vi "CalculatePattern.vi"(4 "Patterns":T2, 5 "error in (no error)":errorcluster, 6 "Colour Set":T1, 8 "NeoPixel Ring in":T1) -> (0 "error out":errorcluster, 2 "NeoPixel Ring out":T1)   [LabVIEW 2020, in "CTI-Scratchpad.lvlib"]
uses:
  CTI-Scratchpad.lvlib
  NeoPixelRingPatterns.ctl
panel:
  # "Input"
  # "Output"
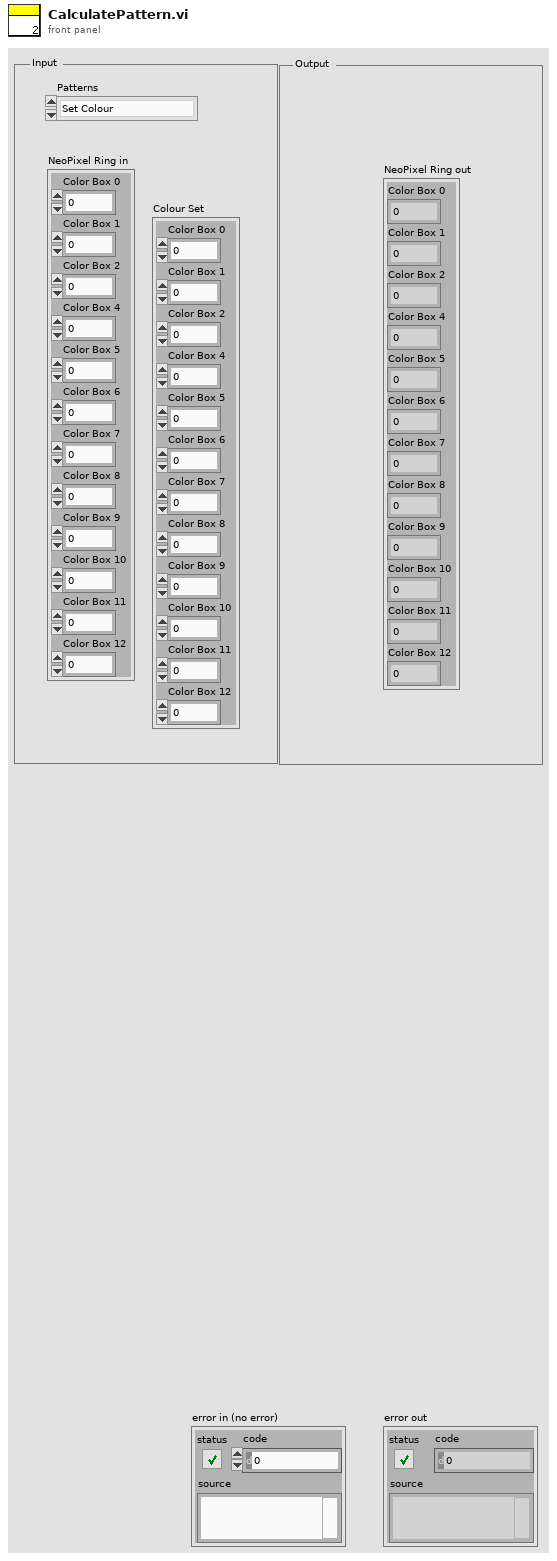
[diagram p1: front panel]
types:
  T1 = cluster{"Color Box 0":u32, "Color Box 1":u32, "Color Box 2":u32, "Color Box 4":u32, "Color Box 5":u32, "Color Box 6":u32, "Color Box 7":u32, "Color Box 8":u32, "Color Box 9":u32, "Color Box 10":u32, "Color Box 11":u32, "Color Box 12":u32}
  T2 = typedef "CTI-Scratchpad.lvlib/NeoPixelRingPatterns.ctl" = enum16{"Set Colour", "ColorWipe", "TheatreChase", "Rainbow"}
  T3 = cluster{"[0]":u32, "[1]":u32, "[2]":u32, "[3]":u32, "[4]":u32, "[5]":u32, "[6]":u32, "[7]":u32, "[8]":u32, "[9]":u32, "[10]":u32, "[11]":u32}
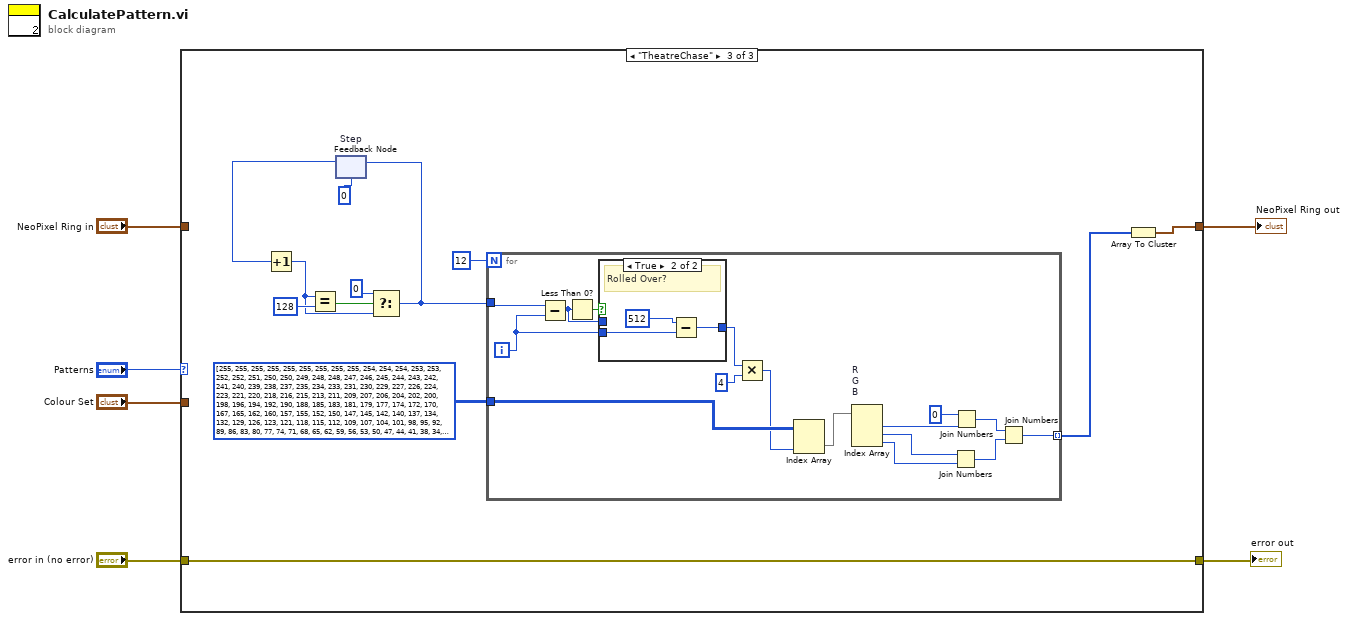
[diagram p0: block diagram]
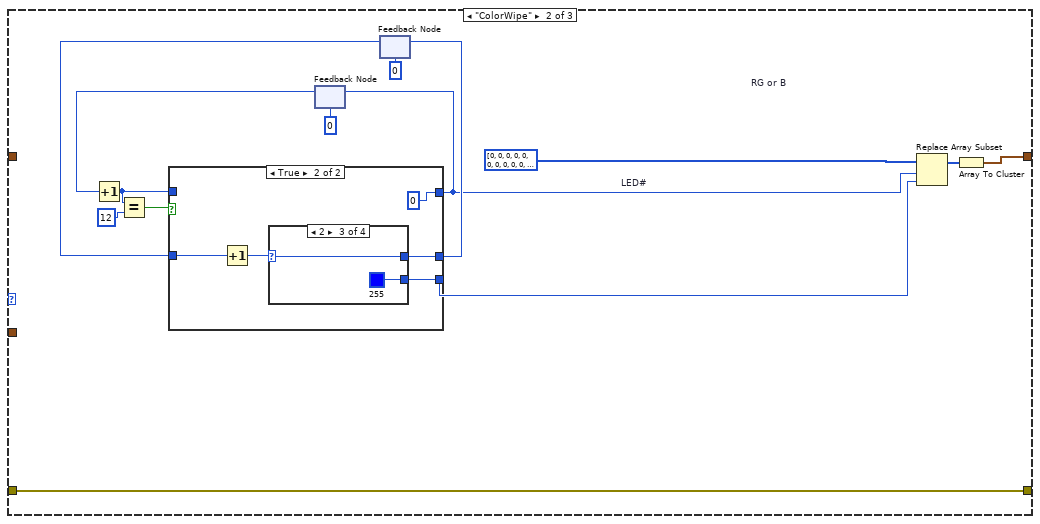
[diagram p3: hidden frame]
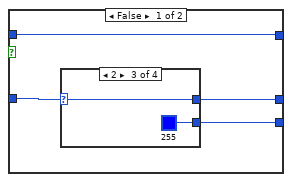
[diagram p4: hidden frame]
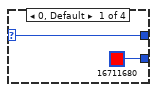
[diagram p5: hidden frame]
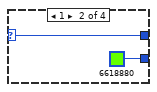
[diagram p6: hidden frame]
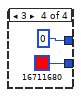
[diagram p7: hidden frame]
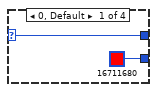
[diagram p8: hidden frame]
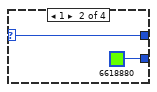
[diagram p9: hidden frame]
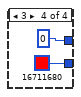
[diagram p10: hidden frame]
diagram:
  n1 = case shown="\"TheatreChase\"" "Patterns" {
    tunnel: "NeoPixel Ring in" -> [_ _ _]
    tunnel: [w8 w10 w56] -> w4
    tunnel: "Colour Set" -> [w8 _ _]
    tunnel: "error in (no error)" -> [w7 w22 w59]
    tunnel: [w7 w22 w59] -> w1
    frame "Set Colour", Default {
    }
    frame "ColorWipe" {
      n2 = feedback #1 "LED#"(u8 0) -> (w19:u8)
      n3 = Increment(x=w19) -> (x+1=w9:u8)
      n4 = Equal?(x=w9, y=u8 12) -> (x = y?=w17:bool)
      n5 = feedback #2 "RG or B"(u8 0) -> (w16:i32)
      n6 = case shown="True" w17 {
        tunnel: w16 -> [w26 w39]
        tunnel: [w23 u8 0] -> w13
        tunnel: [w24 w36] -> w15
        tunnel: [w25 w35] -> w12
        tunnel: w9 -> [w23 _]
        frame False {
          n7 = case shown="2" w26 {
            selector: w26 -> [w27 w29 w31 _]
            tunnel: [w27 w29 w31 u8 0] -> w24
            tunnel: [u32 16711680 ("Color Box 3") u32 6618880 ("Color Box 3") u32 255 ("Color Box 3") u32 16711680 ("Color Box 3")] -> w25
            frame 0, Default {
            }
            frame 1 {
            }
            frame 2 {
            }
            frame 3 {
            }
          }
        }
        frame True {
          n8 = Increment(x=w39) -> (x+1=w37:i32)
          n9 = case shown="2" w37 {
            selector: w37 -> [w40 w42 w44 _]
            tunnel: [w40 w42 w44 u8 0] -> w36
            tunnel: [u32 16711680 ("Color Box 3") u32 6618880 ("Color Box 3") u32 255 ("Color Box 3") u32 16711680 ("Color Box 3")] -> w35
            frame 0, Default {
            }
            frame 1 {
            }
            frame 2 {
            }
            frame 3 {
            }
          }
        }
      }
      n10 = feedback-in #1(w13) -> ()
      n11 = feedback-in #2(w15) -> ()
      n12 = Replace Array Subset(array=u32[] [0, 0, 0, 0, 0, 0, 0, 0, 0, 0, 0, 16777228], new element=w12, index=w13) -> (w11:u32[])
      n13 = Array To Cluster(array=w11) -> (cluster=w10:T3)
    }
    frame "TheatreChase" {
      n14 = feedback #3 "Step"(u16 0) -> (w55:u16)
      n15 = Increment(x=w55) -> (x+1=w52:u16)
      n16 = Equal?(x=w52, y=u16 128) -> (x = y?=w54:bool)
      n17 = Select(t=u16 0, s=w54, f=w52) -> (s? t:f=w48:u16)
      n18 = feedback-in #3(w48) -> ()
      n19 = for {
        N: 12 -> [_]
        tunnel: w48 -> [w75]
        tunnel: u8[][] [[255, 255, 255, 255, 255, 255, 255, 255, 255, 254, 254, 254, 253, 253, 252, 252, 251, 250, 250, 249, 248, 248, 247, 246, 245, 244, 243, 242, 241, 240, 239, 238, 237, 235, 234, 233, 231, 230, 229, 227, 226, 224, 223, 221, 220, 218, 216, 215, 213, 211, 209, 207, 206, 204, 202, 200, 198, 196, 194, 192, 190, 188, 185, 183, 181, 179, 177, 174, 172, 170, 167, 165, 162, 160, 157, 155, 152, 150, 147, 145, 142, 140, 137, 134, 132, 129, 126, 123, 121, 118, 115, 112, 109, 107, 104, 101, 98, 95, 92, 89, 86, 83, 80, 77, 74, 71, 68, 65, 62, 59, 56, 53, 50, 47, 44, 41, 38, 34, 31, 28, 25, 22, 19, 16, 13, 9, 6, 3, 0, 0, 0, 0, 0, 0, 0, 0, 0, 0, 0, 0, 0, 0, 0, 0, 0, 0, 0, 0, 0, 0, 0, 0, 0, 0, 0, 0, 0, 0, 0, 0, 0, 0, 0, 0, 0, 0, 0, 0, 0, 0, 0, 0, 0, 0, 0, 0, 0, 0, 0, 0, 0, 0, 0, 0, 0, 0, 0, 0, 0, 0, 0, 0, 0, 0, 0, 0, 0, 0, 0, 0, 0, 0, 0, 0, 0, 0, 0, 0, 0, 0, 0, 0, 0, 0, 0, 0, 0, 0, 0, 0, 0, 0, 0, 0, 0, 0, 0, 0, 0, 0, 0, 0, 0, 0, 0, 0, 0, 0, 0, 0, 0, 0, 0, 0, 0, 0, 0, 0, 0, 0, 0, 0, 0, 0, 0, 0, 0, 0, 0, 0, 0, 0, 0, 0, 0, 0, 0, 0, 0, 0, 0, 0, 0, 0, 0, 0, 0, 0, 0, 0, 0, 0, 0, 0, 0, 0, 0, 0, 0, 0, 0, 0, 0, 0, 0, 0, 0, 0, 0, 0, 0, 0, 0, 0, 0, 0, 0, 0, 0, 0, 0, 0, 0, 0, 0, 0, 0, 0, 0, 0, 0, 0, 0, 0, 0, 0, 0, 0, 0, 0, 0, 0, 0, 0, 0, 0, 0, 0, 0, 0, 0, 0, 0, 0, 0, 0, 0, 0, 0, 0, 0, 0, 0, 0, 0, 0, 0, 0, 0, 0, 0, 0, 0, 0, 0, 0, 0, 0, 0, 0, 0, 0, 0, 0, 0, 0, 0, 0, 0, 0, 0, 0, 0, 0, 0, 3, 6, 9, 13, 16, 19, 22, 25, 28, 31, 34, 38, 41, 44, 47, 50, 53, 56, 59, 62, 65, 68, 71, 74, 77, 80, 83, 86, 89, 92, 95, 98, 101, 104, 107, 109, 112, 115, 118, 121, 123, 126, 129, 132, 134, 137, 140, 142, 145, 147, 150, 152, 155, 157, 160, 162, 165, 167, 170, 172, 174, 177, 179, 181, 183, 185, 188, 190, 192, 194, 196, 198, 200, 202, 204, 206, 207, 209, 211, 213, 215, 216, 218, 220, 221, 223, 224, 226, 227, 229, 230, 231, 233, 234, 235, 237, 238, 239, 240, 241, 242, 243, 244, 245, 246, 247, 248, 248, 249, 250, 250, 251, 252, 252, 253, 253, 254, 254, 254, 255, 255, 255, 255, 255, 255, 255, 255], [0, 3, 6, 9, 13, 16, 19, 22, 25, 28, 31, 34, 38, 41, 44, 47, 50, 53, 56, 59, 62, 65, 68, 71, 74, 77, 80, 83, 86, 89, 92, 95, 98, 101, 104, 107, 109, 112, 115, 118, 121, 123, 126, 129, 132, 134, 137, 140, 142, 145, 147, 150, 152, 155, 157, 160, 162, 165, 167, 170, 172, 174, 177, 179, 181, 183, 185, 188, 190, 192, 194, 196, 198, 200, 202, 204, 206, 207, 209, 211, 213, 215, 216, 218, 220, 221, 223, 224, 226, 227, 229, 230, 231, 233, 234, 235, 237, 238, 239, 240, 241, 242, 243, 244, 245, 246, 247, 248, 248, 249, 250, 250, 251, 252, 252, 253, 253, 254, 254, 254, 255, 255, 255, 255, 255, 255, 255, 255, 255, 255, 255, 255, 255, 255, 255, 255, 255, 254, 254, 254, 253, 253, 252, 252, 251, 250, 250, 249, 248, 248, 247, 246, 245, 244, 243, 242, 241, 240, 239, 238, 237, 235, 234, 233, 231, 230, 229, 227, 226, 224, 223, 221, 220, 218, 216, 215, 213, 211, 209, 207, 206, 204, 202, 200, 198, 196, 194, 192, 190, 188, 185, 183, 181, 179, 177, 174, 172, 170, 167, 165, 162, 160, 157, 155, 152, 150, 147, 145, 142, 140, 137, 134, 132, 129, 126, 123, 121, 118, 115, 112, 109, 107, 104, 101, 98, 95, 92, 89, 86, 83, 80, 77, 74, 71, 68, 65, 62, 59, 56, 53, 50, 47, 44, 41, 38, 34, 31, 28, 25, 22, 19, 16, 13, 9, 6, 3, 0, 0, 0, 0, 0, 0, 0, 0, 0, 0, 0, 0, 0, 0, 0, 0, 0, 0, 0, 0, 0, 0, 0, 0, 0, 0, 0, 0, 0, 0, 0, 0, 0, 0, 0, 0, 0, 0, 0, 0, 0, 0, 0, 0, 0, 0, 0, 0, 0, 0, 0, 0, 0, 0, 0, 0, 0, 0, 0, 0, 0, 0, 0, 0, 0, 0, 0, 0, 0, 0, 0, 0, 0, 0, 0, 0, 0, 0, 0, 0, 0, 0, 0, 0, 0, 0, 0, 0, 0, 0, 0, 0, 0, 0, 0, 0, 0, 0, 0, 0, 0, 0, 0, 0, 0, 0, 0, 0, 0, 0, 0, 0, 0, 0, 0, 0, 0, 0, 0, 0, 0, 0, 0, 0, 0, 0, 0, 0, 0, 0, 0, 0, 0, 0, 0, 0, 0, 0, 0, 0, 0, 0, 0, 0, 0, 0, 0, 0, 0, 0, 0, 0, 0, 0, 0, 0, 0, 0, 0, 0, 0, 0, 0, 0, 0, 0, 0, 0, 0, 0, 0, 0, 0, 0, 0, 0, 0, 0, 0, 0, 0, 0, 0, 0, 0, 0, 0, 0, 0, 0, 0, 0, 0, 0, 0, 0, 0, 0, 0, 0, 0, 0, 0, 0, 0, 0, 0, 0, 0, 0, 0, 0, 0, 0, 0, 0, 0, 0, 0, 0, 0, 0, 0, 0, 0, 0, 0, 0, 0, 0, 0, 0, 0, 0, 0, 0, 0, 0, 0, 0, 0, 0, 0, 0, 0, 0, 0, 0, 0, 0, 0, 0, 0, 0, 0, 0], [0, 0, 0, 0, 0, 0, 0, 0, 0, 0, 0, 0, 0, 0, 0, 0, 0, 0, 0, 0, 0, 0, 0, 0, 0, 0, 0, 0, 0, 0, 0, 0, 0, 0, 0, 0, 0, 0, 0, 0, 0, 0, 0, 0, 0, 0, 0, 0, 0, 0, 0, 0, 0, 0, 0, 0, 0, 0, 0, 0, 0, 0, 0, 0, 0, 0, 0, 0, 0, 0, 0, 0, 0, 0, 0, 0, 0, 0, 0, 0, 0, 0, 0, 0, 0, 0, 0, 0, 0, 0, 0, 0, 0, 0, 0, 0, 0, 0, 0, 0, 0, 0, 0, 0, 0, 0, 0, 0, 0, 0, 0, 0, 0, 0, 0, 0, 0, 0, 0, 0, 0, 0, 0, 0, 0, 0, 0, 0, 0, 0, 0, 0, 0, 0, 0, 0, 0, 0, 0, 0, 0, 0, 0, 0, 0, 0, 0, 0, 0, 0, 0, 0, 0, 0, 0, 0, 0, 0, 0, 0, 0, 0, 0, 0, 0, 0, 0, 0, 0, 0, 0, 0, 0, 0, 0, 0, 0, 0, 0, 0, 0, 0, 0, 0, 0, 0, 0, 0, 0, 0, 0, 0, 0, 0, 0, 0, 0, 0, 0, 0, 0, 0, 0, 0, 0, 0, 0, 0, 0, 0, 0, 0, 0, 0, 0, 0, 0, 0, 0, 0, 0, 0, 0, 0, 0, 0, 0, 0, 0, 0, 0, 0, 0, 0, 0, 0, 0, 0, 0, 0, 0, 0, 0, 0, 0, 0, 0, 0, 0, 0, 0, 0, 0, 0, 0, 0, 0, 3, 6, 9, 13, 16, 19, 22, 25, 28, 31, 34, 38, 41, 44, 47, 50, 53, 56, 59, 62, 65, 68, 71, 74, 77, 80, 83, 86, 89, 92, 95, 98, 101, 104, 107, 109, 112, 115, 118, 121, 123, 126, 129, 132, 134, 137, 140, 142, 145, 147, 150, 152, 155, 157, 160, 162, 165, 167, 170, 172, 174, 177, 179, 181, 183, 185, 188, 190, 192, 194, 196, 198, 200, 202, 204, 206, 207, 209, 211, 213, 215, 216, 218, 220, 221, 223, 224, 226, 227, 229, 230, 231, 233, 234, 235, 237, 238, 239, 240, 241, 242, 243, 244, 245, 246, 247, 248, 248, 249, 250, 250, 251, 252, 252, 253, 253, 254, 254, 254, 255, 255, 255, 255, 255, 255, 255, 255, 255, 255, 255, 255, 255, 255, 255, 255, 255, 254, 254, 254, 253, 253, 252, 252, 251, 250, 250, 249, 248, 248, 247, 246, 245, 244, 243, 242, 241, 240, 239, 238, 237, 235, 234, 233, 231, 230, 229, 227, 226, 224, 223, 221, 220, 218, 216, 215, 213, 211, 209, 207, 206, 204, 202, 200, 198, 196, 194, 192, 190, 188, 185, 183, 181, 179, 177, 174, 172, 170, 167, 165, 162, 160, 157, 155, 152, 150, 147, 145, 142, 140, 137, 134, 132, 129, 126, 123, 121, 118, 115, 112, 109, 107, 104, 101, 98, 95, 92, 89, 86, 83, 80, 77, 74, 71, 68, 65, 62, 59, 56, 53, 50, 47, 44, 41, 38, 34, 31, 28, 25, 22, 19, 16, 13, 9, 6, 3]] ("Waveform Graph") -> [w73]
        tunnel: [w65] -> w49 mode=indexing
        i -> [w63]
        n20 = Subtract(x=w75, y=w63) -> (x-y=w64:i32)
        n21 = Less Than 0?(x=w64) -> (x < 0?=w74:bool)
        n22 = case shown="True" w74 {
          tunnel: w63 -> [_ w78]
          tunnel: [w76 w77] -> w61
          tunnel: w64 -> [w76 _]
          frame False {
          }
          frame True {
            # "Rolled Over?"
            n23 = Subtract(x=u16 512 ("y"), y=w78) -> (x-y=w77:i32)
          }
        }
        n24 = Multiply(x=w61, y=4 ("x")) -> (x*y=w60:i32)
        n25 = Index Array(array=w73, index (col)=w60) -> (element=w66:u8[])  [unwired: 1 in]
        n26 = Index Array "R\nG\nB"(array=w66) -> (element #1=w72:u8, element #2=w71:u8, element #3=w70:u8)  [unwired: 3 in]
        n27 = Join Numbers(hi=w71, lo=w70) -> ((hi.lo)=w68:u16)
        n28 = Join Numbers(hi=u8 0, lo=w72) -> ((hi.lo)=w69:u16)
        n29 = Join Numbers(hi=w69, lo=w68) -> ((hi.lo)=w65:u32)
      }
      n30 = Array To Cluster(array=w49) -> (cluster=w56:T3)
    }
  }
  "error out" <- w1
  "NeoPixel Ring out" <- w4
